vi "JAPCallTypes.vi"(8 "error in (no error)":errorcluster, 9 "Data Type":string, 11 "JAPCinit":refnum<class "RADEBase.lvclass">) -> (0 "error out":errorcluster, 2 "JAPCout":string, 3 "JAPCexit":refnum<class "RADEBase.lvclass">)   [LabVIEW 2014]
uses:
  <userlib>/_RADE/RIO/RADEBase/classes/RADEBase/RADEBase.lvclass
  <userlib>/_RADE/RIO/JAPC/classes/JSubscribe/JSubscribe.lvclass
  <userlib>/_RADE/RIO/JAPC/classes/JSubscribe/JAPCSubscribe.vi
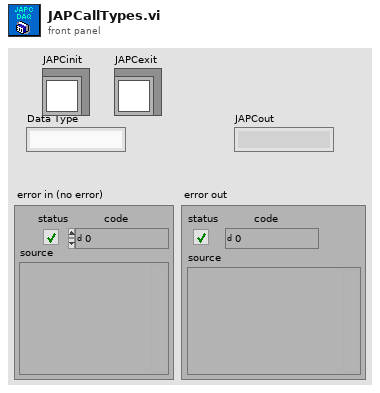
[diagram p1: front panel]
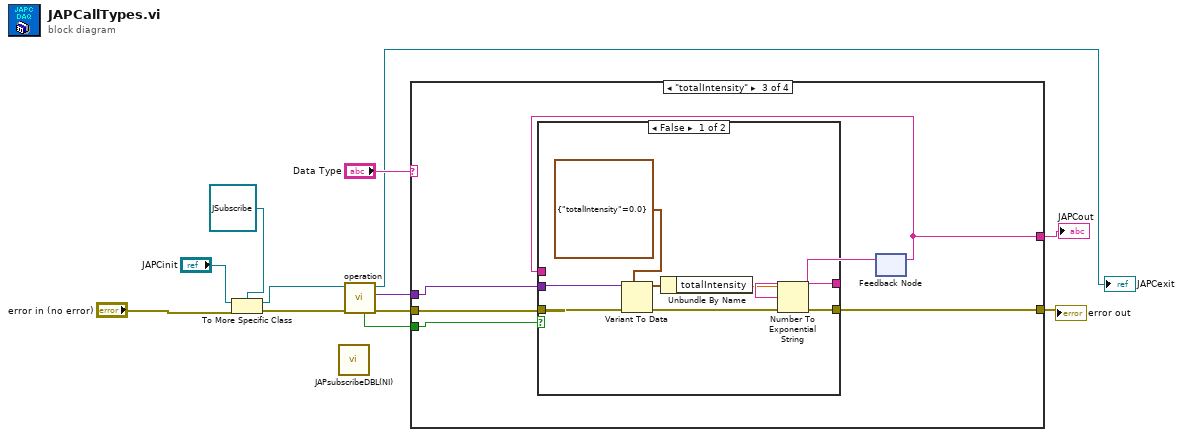
[diagram p0: block diagram]
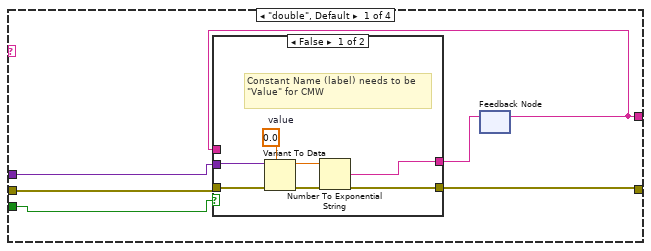
[diagram p2: hidden frame]
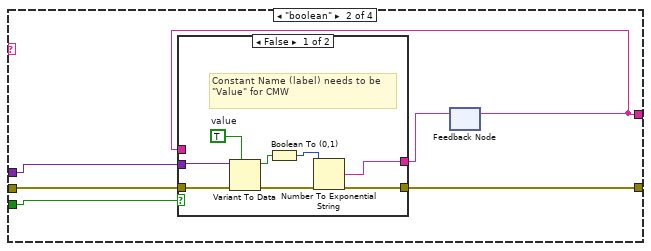
[diagram p4: hidden frame]
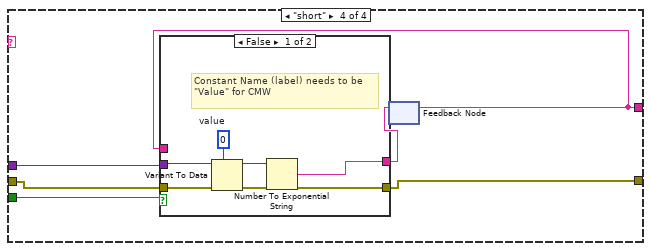
[diagram p7: hidden frame]
diagram:
  n1 = To More Specific Class(target class=refnum<class "JSubscribe.lvclass"> refnum ("JAPBdblIN"), reference="JAPCinit", error in="error in (no error)") -> (specific class reference=w7:refnum<class "JSubscribe.lvclass">, error out=w6:errorcluster)
  n2 = call "JAPsubscribeDBL(NI).vi"() -> ()  [unwired: 9 in, 3 out]
  n3 = call-poly <userlib>:"operation.vi"("error in (no error)"=w6, "Object in"=w7) -> ("error out"=w5:errorcluster, "Data"=w3:variant, "Object out"=→"JAPCexit":refnum<class "JSubscribe.lvclass">, "Timeout?"=w2:bool)  [unwired: 4 in, 2 out]
  n4 = case shown="\"totalIntensity\"" "Data Type" {
    tunnel: w5 -> [w18 w32 w44 w61]
    tunnel: [w16 w27 w46 w59] -> w11
    tunnel: [w14 w28 w42 w57] -> w10
    tunnel: w3 -> [w13 w31 w45 w60]
    tunnel: w2 -> [w17 w30 w43 w62]
    frame "double", Default {
      n5 = feedback #1() -> (w14:string)  [unwired: 1 in]
      n6 = case shown="False" w17 {
        tunnel: w18 -> [w24 w26]
        tunnel: [w23 w26] -> w16
        tunnel: w13 -> [w19 _]
        tunnel: [w21 w25] -> w15
        tunnel: w14 -> [_ w25]
        frame False {
          w20 = 0.0  # value
          # "Constant Name (label) needs to be \"Value\" for CMW"
          n7 = Variant To Data(error in=w24, type=w20, Variant=w19) -> (data=w22:dbl, error out=w23:errorcluster)
          n8 = Number To Exponential String(number=w22) -> (E-format string=w21:string)  [unwired: 3 in]
        }
        frame True {
          # "Subscription Timed Out"
        }
      }
      n9 = feedback-in #1(w15) -> ()
    }
    frame "boolean" {
      n10 = feedback #2() -> (w28:string)  [unwired: 1 in]
      n11 = case shown="False" w30 {
        tunnel: w32 -> [w39 w41]
        tunnel: [w37 w41] -> w27
        tunnel: w31 -> [w38 _]
        tunnel: [w36 w40] -> w29
        tunnel: w28 -> [_ w40]
        frame False {
          w35 = TRUE  # value
          # "Constant Name (label) needs to be \"Value\" for CMW"
          n12 = Variant To Data(error in=w39, type=w35, Variant=w38) -> (data=w33:bool, error out=w37:errorcluster)
          n13 = Boolean To (0,1)(Boolean=w33) -> (0, 1=w34:i16)
          n14 = Number To Exponential String(number=w34) -> (E-format string=w36:string)  [unwired: 3 in]
        }
        frame True {
          # "Subscription Timed Out"
        }
      }
      n15 = feedback-in #2(w29) -> ()
    }
    frame "totalIntensity" {
      n16 = feedback #3() -> (w42:string)  [unwired: 1 in]
      n17 = case shown="False" w43 {
        tunnel: w44 -> [w54 w56]
        tunnel: [w52 w56] -> w46
        tunnel: w45 -> [w53 _]
        tunnel: [w51 w55] -> w47
        tunnel: w42 -> [_ w55]
        frame False {
          n18 = Variant To Data(error in=w54, type=cluster{"totalIntensity":sgl} {"totalIntensity"=0.0}, Variant=w53) -> (data=w50:cluster{"totalIntensity":sgl}, error out=w52:errorcluster)
          n19 = Unbundle By Name(w50) -> ("totalIntensity"=w48:sgl)
          n20 = Number To Exponential String(number=w48) -> (E-format string=w51:string)  [unwired: 3 in]
        }
        frame True {
          # "Subscription Timed Out"
        }
      }
      n21 = feedback-in #3(w47) -> ()
    }
    frame "short" {
      n22 = feedback #4() -> (w57:string)  [unwired: 1 in]
      n23 = case shown="False" w62 {
        tunnel: w61 -> [w68 w70]
        tunnel: [w66 w70] -> w59
        tunnel: w60 -> [w67 _]
        tunnel: [w64 w69] -> w58
        tunnel: w57 -> [_ w69]
        frame False {
          w63 = i16 0  # value
          # "Constant Name (label) needs to be \"Value\" for CMW"
          n24 = Variant To Data(error in=w68, type=w63, Variant=w67) -> (data=w65:i16, error out=w66:errorcluster)
          n25 = Number To Exponential String(number=w65) -> (E-format string=w64:string)  [unwired: 3 in]
        }
        frame True {
          # "Subscription Timed Out"
        }
      }
      n26 = feedback-in #4(w58) -> ()
    }
  }
  "error out" <- w11
  "JAPCout" <- w10
